vi "Loop Async.vi"(11 "ChannelService in":refnum<class "ChannelService.lvclass">) -> ()   [LabVIEW 2020, in "Vecto.lvlib" / "ChannelService.lvclass"]
uses:
  ChannelService.lvclass
  ChannelService.lvclass/ChannelService.ctl
  Loop Data.ctl
  lv-promises/Promises/Promise/Promise.lvclass
  GroupValue/GroupAbstractValue.lvclass
  Group Config/Group Config.lvclass
  Group/Group.lvclass
  GroupsAbstractValue/GroupsAbstractValue.lvclass
  EventLoggingService/EventLoggingService.lvclass
  Event Level.ctl
  Vecto.lvlib
  ChannelValue/DoubleChannelValue.lvclass
  Channel DBL/Channel DBL.lvclass
  Group DBL/Group DBL.lvclass
  Group STR/Group STR.lvclass
  Channel STR/Channel STR.lvclass
  StringChannelValue/StringChannelValue.lvclass
  C:/dev/lv20CE/relink/lv-promises/Promises/Value/Value.lvclass
  C:/dev/lv20CE/relink/lv-vecto/Vecto/GroupValue/GroupAbstractValue.lvclass
  C:/dev/lv20CE/relink/lv-vecto/Vecto/GroupsAbstractValue/GroupsAbstractValue.lvclass
  Group BOOL/Group BOOL.lvclass
  Channel BOOL/Channel BOOL.lvclass
  BoolChannelValue/BoolChannelValue.lvclass
  C:/dev/lv20CE/relink/lv-vecto/Vecto/ChannelValue/DoubleChannelValue.lvclass
  C:/dev/lv20CE/relink/lv-vecto/Vecto/StringChannelValue/StringChannelValue.lvclass
  C:/dev/lv20CE/relink/lv-vecto/Vecto/BoolChannelValue/BoolChannelValue.lvclass
panel:
  out "Last Created Group":string
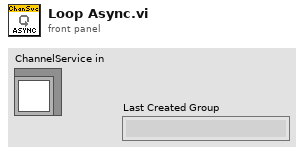
[diagram p1: front panel]
types:
  T1 = typedef "Vecto.lvlib/ChannelService.lvclass/Loop Data.ctl" = cluster{"Groups":refnum<class "Group.lvclass">[], "Channel Group Map":map{string, i32}, "Group Map":map{string, i32}}
  T2 = typedef "Vecto.lvlib/Event Level.ctl" = enum16{"Debug", "Info", "Warning", "Error"}
  T3 = typedef "VectoConfig.lvlib/Group Data Type.ctl" = enum16{"Double", "String", "Bool"}
  T4 = typedef "Vecto.lvlib/ChannelService.lvclass/Lookup Type.ctl" = enum16{"Name", "Node", "Pattern"}
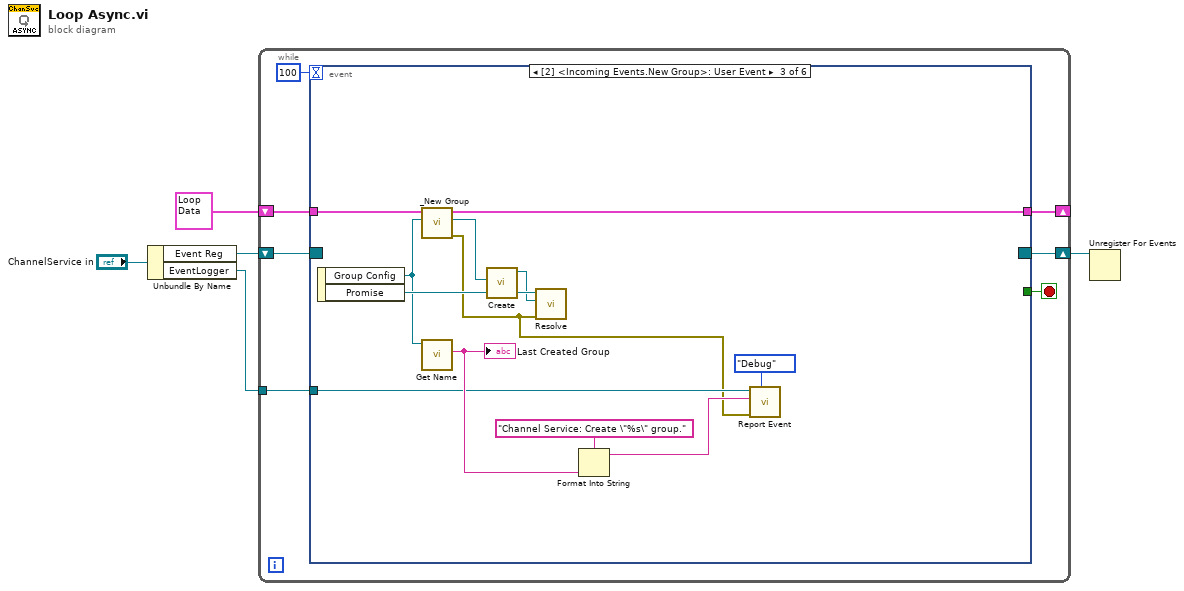
[diagram p0: block diagram]
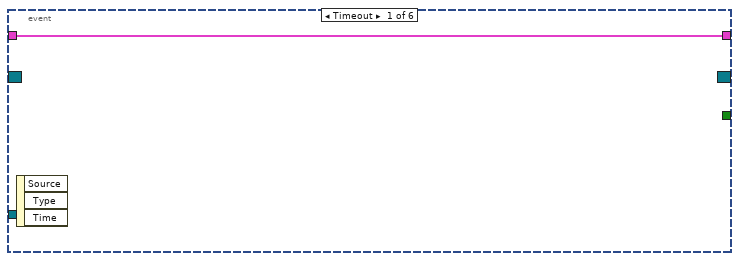
[diagram p2: hidden frame]
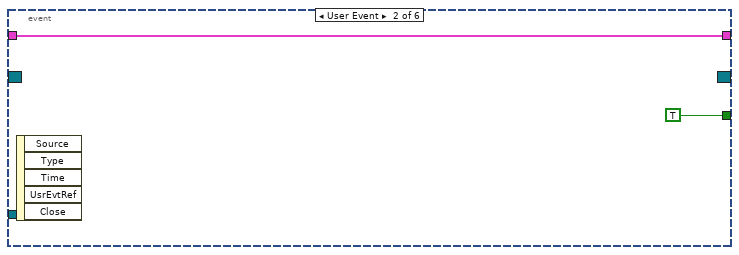
[diagram p3: hidden frame]
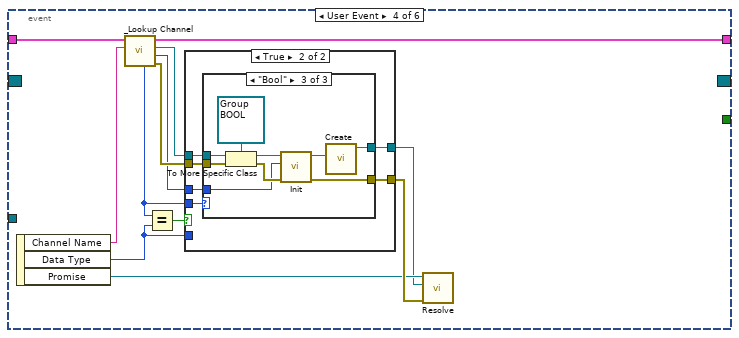
[diagram p4: hidden frame]
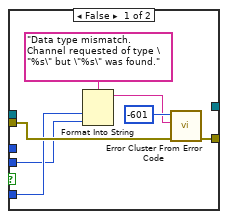
[diagram p5: hidden frame]
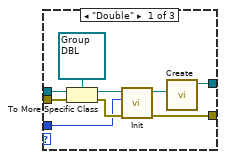
[diagram p6: hidden frame]
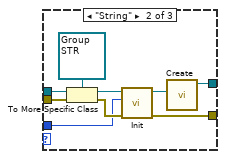
[diagram p7: hidden frame]
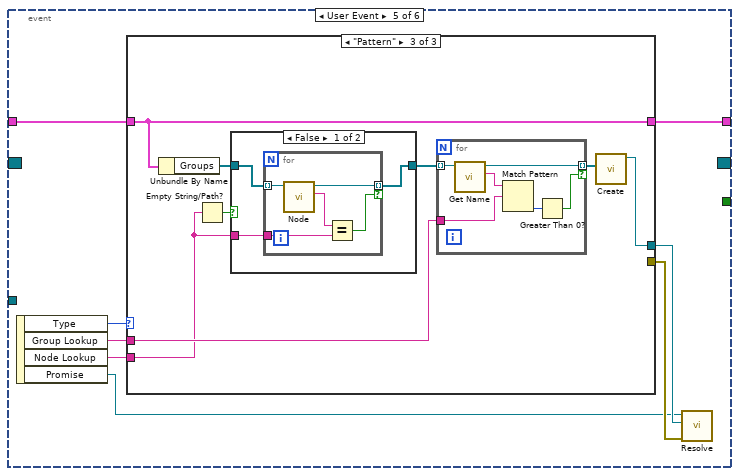
[diagram p8: hidden frame]
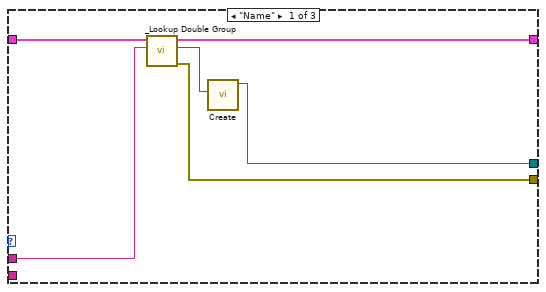
[diagram p9: hidden frame]
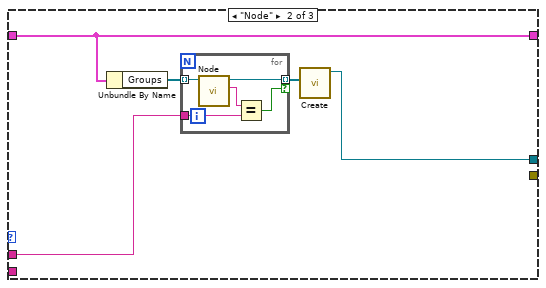
[diagram p10: hidden frame]
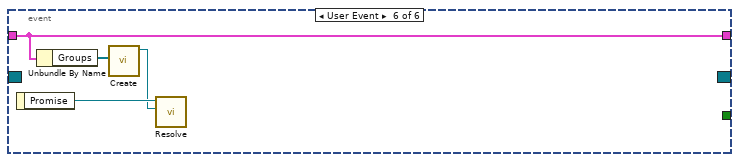
[diagram p12: hidden frame]
diagram:
  n1 = Unbundle By Name("ChannelService in") -> ("Event Reg"=w4:refnum<event-registration>, "EventLogger"=w1:refnum<class "EventLoggingService.lvclass">)
  n2 = while {
    shift-right: [w8] -> w2
    shift-left: w4 -> [w12]
    shift-right: [w9] -> _
    shift-left: T1 {"Groups"=[], "Channel Group Map"={}, "Group Map"={}} ("Loop Data") -> [w10]
    tunnel: w1 -> [w6]
    stop <- w7 stop-if-true
    n3 = event shown="[2] <Incoming Events.New Group>: User Event" {
      selector: w12 -> [_ _ _ _ _ _]
      dyn-events: [_ _ _ _ _ _] -> w8
      timeout: 100 -> [_ _ _ _ _ _]
      tunnel: w10 -> [w13 w15 w27 w37 w86 w130]
      tunnel: [_ TRUE _ _ _ _] -> w7
      tunnel: [w13 w15 w24 w35 w85 w130] -> w9
      tunnel: w6 -> [_ _ w19 _ _ _]
      event Timeout {
        n4 = event-data() -> ()  [unwired: 1 in, 3 out]
      }
      event User Event {
        n5 = event-data() -> ()  [unwired: 1 in, 5 out]
      }
      event User Event {
        n6 = event-data() -> ("Group Config"=w23:refnum<class "Group Config.lvclass">, "Promise"=w26:refnum<class "Promise.lvclass">)  [unwired: 1 in]
        n7 = call "_New Group.vi"("Group Config"=w23, "Loop Data in"=w27) -> ("error out"=w16:errorcluster, "Group"=w22:refnum<class "Group.lvclass">, "Loop Data"=w24:T1)  [unwired: 7 in]
        n8 = call "Get Name.vi"("Group Config in"=w23) -> ("Name"=w20:string)  [unwired: 8 in, 2 out]
        "Last Created Group" <- w20
        n9 = call "Create.vi"("Group"=w22) -> ("GroupValue out"=w25:refnum<class "GroupAbstractValue.lvclass">)  [unwired: 10 in]
        n10 = call "Resolve.vi"("error in (no error)"=w16, "Result"=w25, "Promise in"=w26) -> ()  [unwired: 7 in, 2 out]
        n11 = Format Into String(format string="Channel Service: Create \"%s\" group.", w20) -> (resulting string=w18:string)  [unwired: 2 in, 1 out]
        n12 = call "Report Event.vi"("Event Level (Info)"=Event_Level."Debug", "error in (no error)"=w16, "Message"=w18, "EventLoggingService in"=w19) -> ()  [unwired: 6 in, 2 out]
      }
      event User Event {
        n13 = event-data() -> ("Channel Name"=w34:string, "Data Type"=w28:T3, "Promise"=w36:refnum<class "Promise.lvclass">)  [unwired: 1 in]
        n14 = call "_Lookup Channel.vi"("Channel Name"=w34, "Loop Data 2"=w37) -> ("error out"=w38:errorcluster, "Index"=w30:i32, "Group"=w31:refnum<class "Group.lvclass">, "Loop Data 3"=w35:T1, "Data Type"=w32:T3)  [unwired: 5 in]
        n15 = Equal?(x=w32, y=w28) -> (x = y?=w33:bool)
        n16 = case shown="True" w33 {
          tunnel: w32 -> [w41 w52]
          tunnel: w31 -> [_ w51]
          tunnel: w30 -> [_ w50]
          tunnel: w38 -> [w44 w49]
          tunnel: [w46 w48] -> w39
          tunnel: [_ w47] -> w29
          tunnel: w28 -> [w42 _]
          frame False {
            n17 = Format Into String(format string="Data type mismatch. Channel requested of type \"%s\" but \"%s\" was found.", w42, w41) -> (resulting string=w40:string)  [unwired: 2 in, 1 out]
            n18 = call <vilib>:"Error Cluster From Error Code.vi"("error in (no error)"=w44, "error message (\"\")"=w40, "error code (0)"=-601) -> ("error out"=w46:errorcluster)  [unwired: 6 in]
          }
          frame True {
            n19 = case shown="\"Bool\"" w52 {
              tunnel: w51 -> [w60 w69 w78]
              tunnel: w50 -> [w56 w65 w74]
              tunnel: w49 -> [w57 w66 w75]
              tunnel: [w54 w63 w72] -> w48
              tunnel: [w53 w62 w71] -> w47
              frame "Double" {
                n20 = To More Specific Class(target class=refnum<class "Group DBL.lvclass"> refnum ("Group"), reference=w60, error in=w57) -> (specific class reference=w59:refnum<class "Group DBL.lvclass">, error out=w61:errorcluster)
                n21 = call "Init.vi"("error in (no error)"=w61, "Channel Index"=w56, "Group"=w59) -> ("error out"=w54:errorcluster, "Channel out"=w55:refnum<class "Channel DBL.lvclass">)  [unwired: 7 in]
                n22 = call "Create.vi"("Channel"=w55) -> ("ChannelValue out"=w53:refnum<class "DoubleChannelValue.lvclass">)  [unwired: 10 in]
              }
              frame "String" {
                n23 = To More Specific Class(target class=refnum<class "Group STR.lvclass"> refnum ("Group"), reference=w69, error in=w66) -> (specific class reference=w68:refnum<class "Group STR.lvclass">, error out=w70:errorcluster)
                n24 = call "Init.vi"("error in (no error)"=w70, "Index"=w65, "Group"=w68) -> ("error out"=w63:errorcluster, "StringChannel out"=w64:refnum<class "Channel STR.lvclass">)  [unwired: 7 in]
                n25 = call "Create.vi"("Channel"=w64) -> ("ChannelValue out"=w62:refnum<class "StringChannelValue.lvclass">)  [unwired: 10 in]
              }
              frame "Bool" {
                n26 = To More Specific Class(target class=refnum<class "Group BOOL.lvclass"> refnum ("Group"), reference=w78, error in=w75) -> (specific class reference=w77:refnum<class "Group BOOL.lvclass">, error out=w79:errorcluster)
                n27 = call "Init.vi"("error in (no error)"=w79, "Index"=w74, "Group"=w77) -> ("error out"=w72:errorcluster, "Channel BOOL out"=w73:refnum<class "Channel BOOL.lvclass">)  [unwired: 7 in]
                n28 = call "Create.vi"("Channel"=w73) -> ("BoolChannelValue out"=w71:refnum<class "BoolChannelValue.lvclass">)  [unwired: 10 in]
              }
            }
          }
        }
        n29 = call "Resolve.vi"("error in (no error)"=w39, "Result"=w29, "Promise in"=w36) -> ()  [unwired: 7 in, 2 out]
      }
      event User Event {
        n30 = event-data() -> ("Type"=w82:T4, "Group Lookup"=w84:string, "Node Lookup"=w80:string, "Promise"=w81:refnum<class "Promise.lvclass">)  [unwired: 1 in]
        n31 = case shown="\"Pattern\"" w82 {
          tunnel: [w93 _ _] -> w87
          tunnel: w86 -> [w92 w96 w109]
          tunnel: [w91 w96 w109] -> w85
          tunnel: w84 -> [w90 w94 w108]
          tunnel: [w88 w97 w110] -> w83
          tunnel: w80 -> [_ _ w105]
          frame "Name" {
            n32 = call "_Lookup Double Group.vi"("Group Name"=w90, "Loop Data in"=w92) -> ("error out"=w93:errorcluster, "Group"=w89:refnum<class "Group.lvclass">, "Loop Data"=w91:T1)  [unwired: 7 in]
            n33 = call "Create.vi"("Group"=w89) -> ("GroupValue out"=w88:refnum<class "GroupAbstractValue.lvclass">)  [unwired: 10 in]
          }
          frame "Node" {
            n34 = Unbundle By Name(w96) -> ("Groups"=w95:refnum<class "Group.lvclass">[])
            n35 = for {
              tunnel: w95 -> [w103] mode=indexing
              tunnel: w94 -> [w102]
              tunnel: [w100] -> w98 mode=indexing if=w99
              n36 = call "Node.vi"("Group in"=w103) -> ("Node"=w101:string, "Group out"=w100:refnum<class "Group.lvclass">)  [unwired: 8 in, 1 out]
              n37 = Equal?(x=w101, y=w102) -> (x = y?=w99:bool)
            }
            n38 = call "Create.vi"("Groups"=w98) -> ("GroupsAbstractValue out"=w97:refnum<class "GroupsAbstractValue.lvclass">)  [unwired: 10 in]
          }
          frame "Pattern" {
            n39 = Unbundle By Name(w109) -> ("Groups"=w107:refnum<class "Group.lvclass">[])
            n40 = Empty String/Path?(string/path=w105) -> (empty?=w106:bool)
            n41 = case shown="False" w106 {
              tunnel: w107 -> [w114 w120]
              tunnel: w105 -> [w112 _]
              tunnel: [w113 w120] -> w104
              frame False {
                n42 = for {
                  tunnel: w114 -> [w119] mode=indexing
                  tunnel: [w118] -> w113 mode=indexing if=w115
                  tunnel: w112 -> [w117]
                  n43 = call "Node.vi"("Group in"=w119) -> ("Node"=w116:string, "Group out"=w118:refnum<class "Group.lvclass">)  [unwired: 8 in, 1 out]
                  n44 = Equal?(x=w116, y=w117) -> (x = y?=w115:bool)
                }
              }
              frame True {
              }
            }
            n45 = for {
              tunnel: w104 -> [w126] mode=indexing
              tunnel: w108 -> [w123]
              tunnel: [w125] -> w111 mode=indexing if=w121
              n46 = call "Get Name.vi"("Group in"=w126) -> ("Name"=w124:string, "Group out"=w125:refnum<class "Group.lvclass">)  [unwired: 8 in, 1 out]
              n47 = Match Pattern(string=w124, regular expression=w123) -> (offset past match=w122:i32)  [unwired: 1 in, 3 out]
              n48 = Greater Than 0?(x=w122) -> (x > 0?=w121:bool)
            }
            n49 = call "Create.vi"("Groups"=w111) -> ("GroupsAbstractValue out"=w110:refnum<class "GroupsAbstractValue.lvclass">)  [unwired: 10 in]
          }
        }
        n50 = call "Resolve.vi"("error in (no error)"=w87, "Result"=w83, "Promise in"=w81) -> ()  [unwired: 7 in, 2 out]
      }
      event User Event {
        n51 = event-data() -> ("Promise"=w128:refnum<class "Promise.lvclass">)  [unwired: 1 in]
        n52 = Unbundle By Name(w130) -> ("Groups"=w129:refnum<class "Group.lvclass">[])
        n53 = call "Create.vi"("Groups"=w129) -> ("GroupsAbstractValue out"=w127:refnum<class "GroupsAbstractValue.lvclass">)  [unwired: 10 in]
        n54 = call "Resolve.vi"("Result"=w127, "Promise in"=w128) -> ()  [unwired: 8 in, 2 out]
      }
    }
  }
  n55 = Unregister For Events(event registration refnum=w2) -> ()  [unwired: 1 in, 1 out]
